vi "InitMeaSplitInfo2.vi"(8 "error in (no error)":errorcluster, 10 "Measurement Signals":refnum<k21>[](array[refnum])=["VLKAW_LKAWState_enum\n:memory:.DAQLists", "VOUTP_EPSCtrlSta_enum\n:memory:.DAQLists", "VVHC_SASAngle_deg\n:memory:.DAQLists", "VVHC_VehSpd_kph__S1_\n:memory:.DAQLists", "VVHC_VehSpd_kph__S2_\n:memory:.DAQLists", "VVHC_YawRate_degps\n:memory:.DAQLists", "VCAS_LatFcnSlct_enum\n:memory:.DAQLists", "VLKAW_DistTatY2RefBasL_m\n:memory:.DAQLists", "VLKAW_DistTatY2RefBasR_m__S1_\n:memory:.DAQLists", "VLKAW_DistTatY2RefBasR_m__S2_\n:memory:.DAQLists", "VOUTP_StrAngReq_deg\n:memory:.DAQLists", "VTTD_LKAC0VehWdR_flg\n:memory:.DAQLists", "VTTD_LKAWDvrStrFgt_flg\n:memory:.DAQLists", "VTTD_LKAWVehToLftLn_flg\n:memory:.DAQLists", "VLFS_TLCL_s\n:memory:.DAQLists", "VLFS_TLCR_s__S1_\n:memory:.DAQLists", "VLFS_TLCR_s__S2_\n:memory:.DAQLists", "VLKAW_LKAAssist_flg\n:memory:.DAQLists", "VLKAW_LKAWWarning_enum\n:memory:.DAQLists", "VTTD_LKAWR2LLn_flg\n:memory:.DAQLists", "VLFS_LaneC0R_m\n:memory:.DAQLists", "VLFS_LaneC1R_rad__S1_\n:memory:.DAQLists", "VLFS_LaneC1R_rad__S2_\n:memory:.DAQLists", "VLFS_LaneC2R_rat\n:memory:.DAQLists", "VLFS_LaneC3R_rat__S1_\n:memory:.DAQLists", "VLFS_LaneC3R_rat__S2_\n:memory:.DAQLists", "VEGD_YawRateEst_degps\n:memory:.DAQLists", "VLFS_LaneC0L_m__S1_\n:memory:.DAQLists", "VLFS_LaneC0L_m__S2_\n:memory:.DAQLists", "VLFS_LaneC1L_rad\n:memory:.DAQLists", "VLFS_LaneC2L_rat__S1_\n:memory:.DAQLists", "VLFS_LaneC2L_rat__S2_\n:memory:.DAQLists", "VDCT_PredLatY_m\n:memory:.DAQLists", "VDCT_StrAngReqNoFltT_deg__S1_\n:memory:.DAQLists", "VDCT_StrAngReqNoFltT_deg__S2_\n:memory:.DAQLists", "VDCT_YawRate_degps\n:memory:.DAQLists", "VLKAW_TargetLatY_m__S1_\n:memory:.DAQLists", "VLKAW_TargetLatY_m__S2_\n:memory:.DAQLists", "VLFS_CenterLineC0_m\n:memory:.DAQLists", "VLFS_CenterLineC1_rad__S1_\n:memory:.DAQLists", "VLFS_CenterLineC1_rad__S2_\n:memory:.DAQLists", "VLFS_CenterLineC2_rat\n:memory:.DAQLists", "VLFS_CenterLineC3_rat__S1_\n:memory:.DAQLists", "VLFS_CenterLineC3_rat__S2_\n:memory:.DAQLists", "VLFS_LeftLaneAvail_flg\n:memory:.DAQLists", "VLFS_RightLaneAvail_flg\n:memory:.DAQLists", "VVHC_LSSWarnTiming_enum\n:memory:.DAQLists", "VDCT_AngCmmdDeact_flg\n:memory:.DAQLists", "VEVS_CameraStatus_enum\n:memory:.DAQLists", "VLKAW_LeftLaneRef_m\n:memory:.DAQLists", "VLKAW_RightLaneRef_m__S1_\n:memory:.DAQLists", "VLKAW_RightLaneRef_m__S2_\n:memory:.DAQLists", "VLKAW_TrajLeftLaneBas_m\n:memory:.DAQLists", "VVHC_LongAccel_mps2\n:memory:.DAQLists", "VLFS_LaneRadiusC_m\n:memory:.DAQLists", "VLKAW_TrajRightLane_m__S1_\n:memory:.DAQLists", "VLKAW_TrajRightLane_m__S2_\n:memory:.DAQLists", "VTTD_LKAC0VehWdL_m\n:memory:.DAQLists", "VTTD_LKAC0VehWdR_m__S1_\n:memory:.DAQLists", "VTTD_LKAC0VehWdR_m__S2_\n:memory:.DAQLists", "VDCT_StrTqAppl_flg\n:memory:.DAQLists", "VDCT_StrTqReq_Nm\n:memory:.DAQLists", "VLKAW_TrajctrLnL_m__S1_\n:memory:.DAQLists", "VLKAW_TrajctrLnL_m__S2_\n:memory:.DAQLists", "VLKAW_TrajctrLnR_m\n:memory:.DAQLists", "VTTD_LKAWNearLaneL_flg\n:memory:.DAQLists", "VTTD_LKAWNearLaneR_flg\n:memory:.DAQLists", "VTTD_LKAWVehToLftLn_m\n:memory:.DAQLists", "VTTD_LKAWVehToRgtLn_m__S1_\n:memory:.DAQLists", "VTTD_LKAWVehToRgtLn_m__S2_\n:memory:.DAQLists", "VHAL_CPU1Load_num\n:memory:.DAQLists", "VHAL_CPU2Load_num\n:memory:.DAQLists", "VLFS_LaneWidthAvail_flg\n:memory:.DAQLists", "VLFS_PreviewLaneRadiusC_m\n:memory:.DAQLists", "VLKAW_LookAheadDist_m\n:memory:.DAQLists", "VLKAW_TrajctrLnMinL_m__S1_\n:memory:.DAQLists", "VLKAW_TrajctrLnMinL_m__S2_\n:memory:.DAQLists", "VLKAW_TrajctrLnMinR_m\n:memory:.DAQLists", "VTTD_LKAMissAsstR_flg\n:memory:.DAQLists", "VTTD_LKAWChkNorm_flg\n:memory:.DAQLists", "VTTD_LKAWTLCChckL_flg\n:memory:.DAQLists", "VTTD_LKAWTLCChckR_flg\n:memory:.DAQLists", "VTTD_LKAWTLCFnlL_s\n:memory:.DAQLists", "VLKAW_StopTraLnInL_flg\n:memory:.DAQLists", "VLKAW_StopTraLnInR_flg\n:memory:.DAQLists", "VLKAW_StopTraLnRSL_flg\n:memory:.DAQLists", "VLKAW_StopTraLnRSR_flg\n:memory:.DAQLists", "VLKAW_TrajctrLnFnlL_m__S1_\n:memory:.DAQLists", "VLKAW_TrajctrLnFnlL_m__S2_\n:memory:.DAQLists", "VLKAW_TrajctrLnFnlR_m\n:memory:.DAQLists", "VTTD_LFCRVIChckPass_flg\n:memory:.DAQLists", "VTTD_LKAInActL_flg\n:memory:.DAQLists", "VTTD_LKAInActR_flg\n:memory:.DAQLists", "VTTD_LKALnPredYL_flg\n:memory:.DAQLists", "VTTD_LKAMissAsstL_flg\n:memory:.DAQLists", "VTTD_LKAWDvrTurning_flg\n:memory:.DAQLists", "VTTD_LKAWTLCFnlR_s__S1_\n:memory:.DAQLists", "VTTD_LKAWTLCFnlR_s__S2_\n:memory:.DAQLists", "VHAL_AccelPedalPosn_pct\n:memory:.DAQLists", "VLKAW_DDWTiming1P_s__S1_\n:memory:.DAQLists", "VLKAW_DDWTiming1P_s__S2_\n:memory:.DAQLists", "VLKAW_DDWTiming2P_s\n:memory:.DAQLists", "VLKAW_DDWTiming3P_s__S1_\n:memory:.DAQLists", "VLKAW_DDWTiming3P_s__S2_\n:memory:.DAQLists", "VLKAW_DistTatY2RefTL_m\n:memory:.DAQLists", "VLKAW_DistTatY2RefTR_m__S1_\n:memory:.DAQLists", "VLKAW_DistTatY2RefTR_m__S2_\n:memory:.DAQLists", "VLKAW_DvrDrwWarn1P_flg\n:memory:.DAQLists", "VLKAW_DvrDrwWarn2P_flg\n:memory:.DAQLists", "VLKAW_DvrDrwWarn3P_flg\n:memory:.DAQLists", "VLKAW_DvrDrwWarnC_flg\n:memory:.DAQLists", "VLKAW_DvrDrwWarn_enum\n:memory:.DAQLists", "VOUTP_LDWSSta_enum\n:memory:.DAQLists", "VTTD_LFCOnCondMet_flg\n:memory:.DAQLists", "VTTD_LKAWSpdInRng_flg\n:memory:.DAQLists", "VVHC_LKAEnableH_flg\n:memory:.DAQLists", "VLFS_LaneWidth_m\n:memory:.DAQLists", "VLFS_NextLaneWidthR_m__S1_\n:memory:.DAQLists", "VLFS_NextLaneWidthR_m__S2_\n:memory:.DAQLists", "VTTD_LDWInActL_flg\n:memory:.DAQLists", "VTTD_LDWInActR_flg\n:memory:.DAQLists", "VTTD_LKAEPSRdy_flg\n:memory:.DAQLists", "VTTD_LKAVeh2LnDis_flg\n:memory:.DAQLists", "VTTD_LKAWDvrHndOnCnfi_flg\n:memory:.DAQLists", "VTTD_LKAWDvrNoStrFgt_flg\n:memory:.DAQLists", "VTTD_LKAWDvrNoTurning_flg\n:memory:.DAQLists", "VTTD_LKAWHndOnCnd_flg\n:memory:.DAQLists", "VTTD_LKAWLaneAvail_flg\n:memory:.DAQLists", "VTTD_LKAWLnCrvEnbl_flg\n:memory:.DAQLists", "VTTD_LKAWLnRefL_m__S1_\n:memory:.DAQLists", "VTTD_LKAWLnRefL_m__S2_\n:memory:.DAQLists", "VTTD_LKAWLnRefR_m\n:memory:.DAQLists", "VTTD_LKAWLnWdth4Act_flg\n:memory:.DAQLists", "VTTD_LKAWNoAEBAct_flg\n:memory:.DAQLists", "VTTD_LKAWNoFCWAct_flg\n:memory:.DAQLists", "VVHC_LatAccel_mps2\n:memory:.DAQLists", "VVHC_YawRateKF_radps__S1_\n:memory:.DAQLists", "VVHC_YawRateKF_radps__S2_\n:memory:.DAQLists"], 11 "DAQList in":refnum<class "DAQList.lvclass">) -> (0 "error out":errorcluster, 3 "DAQList out":refnum<class "DAQList.lvclass">)   [LabVIEW 2019, in "XCP_DaqDtoId.lvlib" / "DAQList.lvclass"]
uses:
  DAQList.lvclass
  TypeDef/MeaSplitInfo2.ctl
  DAQList.lvclass/DAQList.ctl
  TypeDef/Global.vi
  <vilib>/ECUMC/ECUMC.llb/MC Get Prop Meas Data Type.vi
  <resource>/objmgr/xnet.rc
  <vilib>/ECUMC/ECUMC.lvlib
panel:
  out "Engine.Meas Split Info":T1[](array[typedef]) {"Byte Order" items=["Little Endian", "Big Endian"]; "Data Type" items=["Signed", "Unsigned", "IEEE Float", "Byte Array"]}
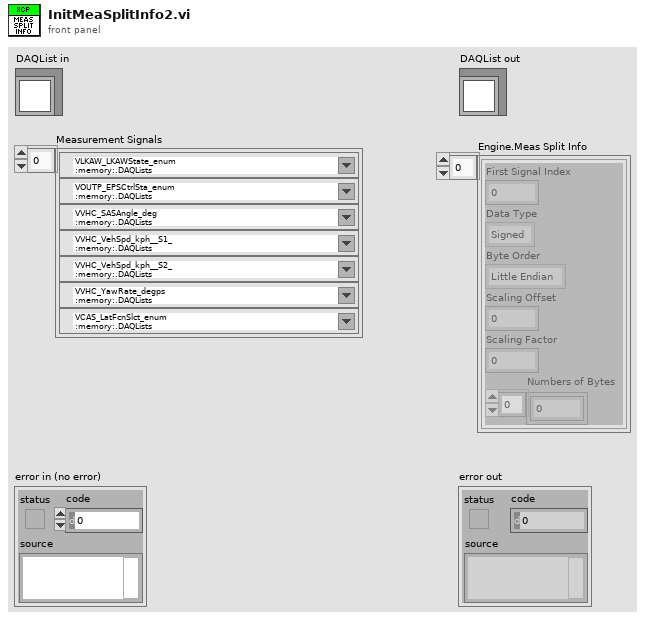
[diagram p1: front panel]
types:
  T1 = typedef "XCP_DaqDtoId.lvlib/DAQList.lvclass/MeaSplitInfo2.ctl" = cluster{"First Signal Index":i32, "Data Type":u32, "Byte Order":u32, "Scaling Offset":dbl, "Scaling Factor":dbl, "Numbers of Bytes":i32[]}
  T2 = typedef "ECUMC.lvlib/MC Reference.ctt" = u32
  T3 = typedef "ECUMC.lvlib/MC Data Type.ctt" = u8
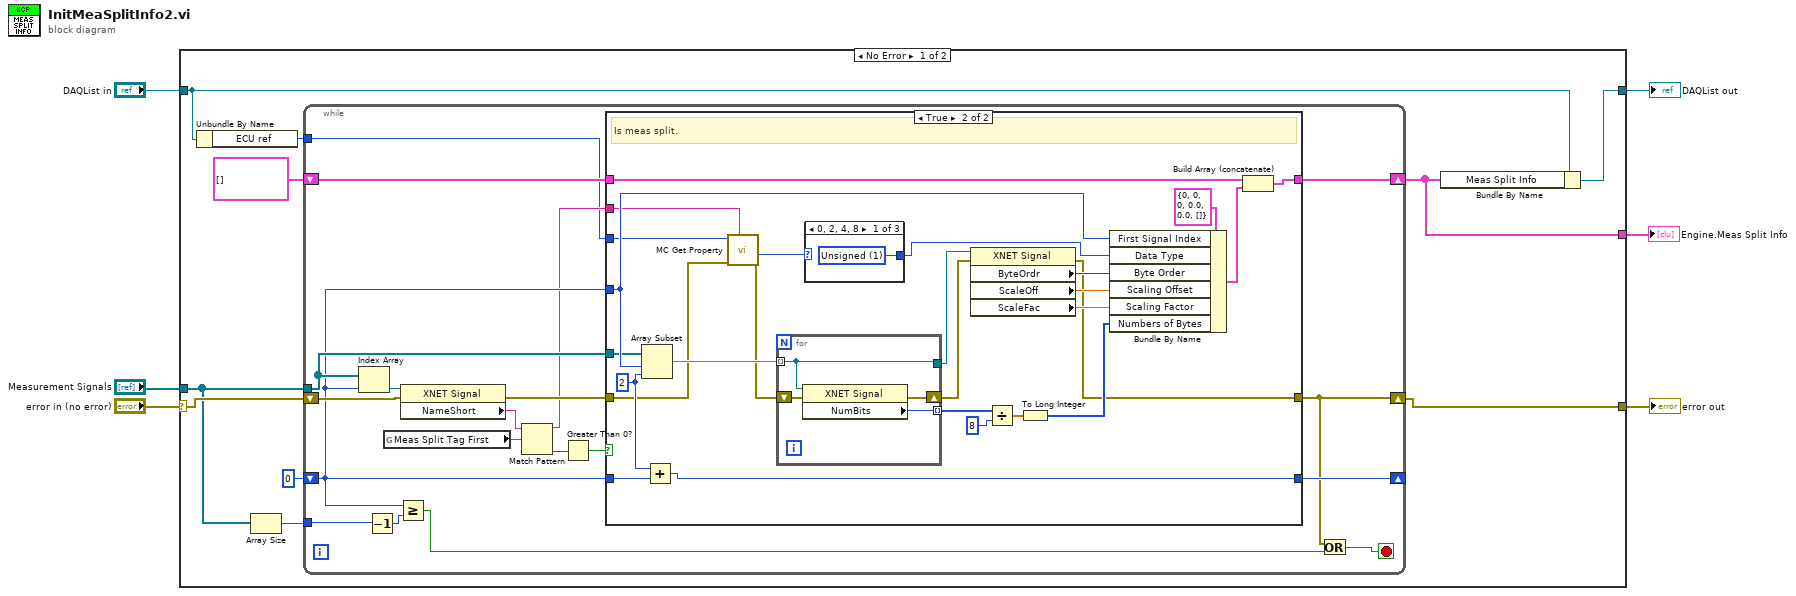
[diagram p0: block diagram]
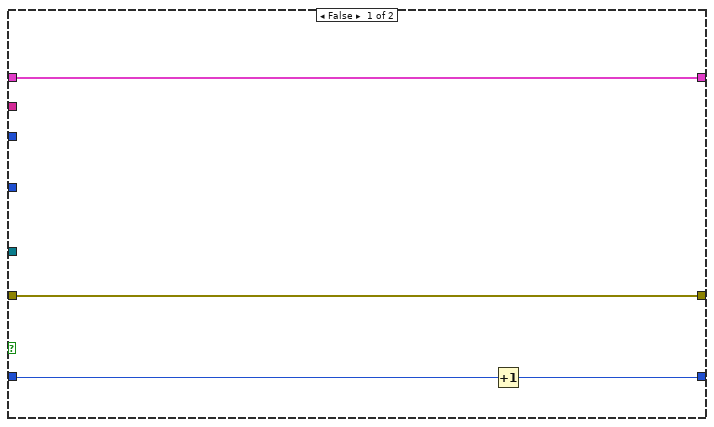
[diagram p2: hidden frame]
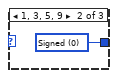
[diagram p3: hidden frame]
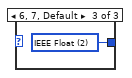
[diagram p4: hidden frame]
diagram:
  n1 = case shown="No Error" "error in (no error)" {
    selector: "error in (no error)" -> [w14 w74]
    tunnel: [w13 w74] -> w5
    tunnel: [w16 w73] -> w3
    tunnel: "DAQList in" -> [w8 w73]
    tunnel: "Measurement Signals" -> [w12 _]
    tunnel: [w9 _] -> w1
    frame No Error {
      n2 = Unbundle By Name(w8) -> ("ECU ref"=w7:T2)
      n3 = Array Size(array=w12) -> (size(s)=w10:i32)
      n4 = while {
        tunnel: w12 -> [w26]
        shift-right: [w28] -> w9
        shift-left: T1[] [] ("Engine.Meas Split Info") -> [w29]
        shift-right: [w21] -> w13
        shift-left: w14 -> [w31]
        shift-right: [w25] -> _
        shift-left: 0 -> [w22]
        tunnel: w10 -> [w24]
        tunnel: w7 -> [w17]
        stop <- w19 stop-if-true
        n5 = Index Array(array=w26, index=w22) -> (element=w27:refnum<k21>)
        n6 = Decrement(x=w24) -> (x-1=w23:i32)
        n7 = global read "Global.vi" "Meas Split Tag First"() -> (w34:string)
        n8 = Greater Or Equal?(x=w22, y=w23) -> (x >= y?=w20:bool)
        n9 = property class="XNET Signal"(reference=w27, error in=w31) -> (error out=w32:errorcluster, "NameShort"=w35:string)  [unwired: 1 out]
        n10 = Match Pattern(string=w35, regular expression=w34) -> (before substring=w18:string, offset past match=w33:i32)  [unwired: 1 in, 2 out]
        n11 = Greater Than 0?(x=w33) -> (x > 0?=w30:bool)
        n12 = case shown="True" w30 {
          tunnel: w22 -> [_ w65]
          tunnel: w32 -> [w38 w41]
          tunnel: [w38 w46] -> w21
          tunnel: w29 -> [w39 w59]
          tunnel: [w39 w58] -> w28
          tunnel: w26 -> [_ w54]
          tunnel: [w37 w62] -> w25
          tunnel: w22 -> [w36 w64]
          tunnel: w18 -> [_ w44]
          tunnel: w17 -> [_ w43]
          frame False {
            n13 = Increment(x=w36) -> (x+1=w37:i32)
          }
          frame True {
            w63 = 2 ("length")
            # "Is meas split."
            n14 = Array Subset(array=w54, index=w65, length=w63) -> (w53:refnum<k21>[])
            n15 = Add(x=w63, y=w64) -> (x+y=w62:i32)
            n16 = call-poly <vilib>:"MC Get Property.vi"("name"=w44, "error in"=w41, "reference in"=w43) -> ("error out"=w40:errorcluster, "meas data type"=w45:T3)  [unwired: 6 in, 1 out]
            n17 = for {
              tunnel: [w71] -> w55 mode=indexing
              shift-right: [w70] -> w50
              shift-left: w40 -> [w72]
              tunnel: w53 -> [w69] mode=indexing
              tunnel: [w69] -> w51
              n18 = property class="XNET Signal"(reference=w69, error in=w72) -> (error out=w70:errorcluster, "NumBits"=w71:u32)  [unwired: 1 out]
            }
            n19 = case shown="0, 2, 4, 8" w45 {
              tunnel: [w66 w67 w68] -> w42
              frame 0, 2, 4, 8 {
                w66 = u32 1 items=["Signed", "Unsigned", "IEEE Float", "Byte Array"] ("Data Type")
              }
              frame 1, 3, 5, 9 {
                w67 = u32 0 items=["Signed", "Unsigned", "IEEE Float", "Byte Array"] ("Data Type")
              }
              frame 6, 7, Default {
                w68 = u32 2 items=["Signed", "Unsigned", "IEEE Float", "Byte Array"] ("Data Type")
              }
            }
            n20 = property class="XNET Signal"(reference=w51, error in=w50) -> (error out=w46:errorcluster, "ByteOrdr"=w49:u32, "ScaleOff"=w48:dbl, "ScaleFac"=w47:dbl)  [unwired: 1 out]
            n21 = Divide(x=w55, y=8) -> (x/y=w56:dbl[])
            n22 = To Long Integer(number=w56) -> (32bit integer=w52:i32[])
            n23 = Bundle By Name(cluster=T1 {"First Signal Index"=0, "Data Type"=0, "Byte Order"=0, "Scaling Offset"=0.0, "Scaling Factor"=0.0, "Numbers of Bytes"=[]} ("Meas Split Info"), "First Signal Index"=w65, "Data Type"=w42, "Byte Order"=w49, "Scaling Offset"=w48, "Scaling Factor"=w47, "Numbers of Bytes"=w52) -> (w61:T1)
            n24 = Build Array (concatenate)(w59, w61) -> (w58:T1[])
          }
        }
        n25 = Or(x=w21, y=w20) -> (x .or. y?=w19:bool)
      }
      n26 = Bundle By Name(cluster=w8, "Meas Split Info"=w9) -> (w16:refnum<class "DAQList.lvclass">)
    }
    frame Error {
    }
  }
  "error out" <- w5
  "DAQList out" <- w3
  "Engine.Meas Split Info" <- w1
